vi "Matches.vi"(8 "error in (no error)":errorcluster, 10 "Actual":variant, 11 "Collection Is Empty in":refnum<class "Collection Is Empty.lvclass">) -> (0 "error out":errorcluster, 2 "Result":bool, 3 "Collection Is Empty out":refnum<class "Collection Is Empty.lvclass">)   [LabVIEW 2017, in "Transparent Assertions.lvlib" / "Collection Is Empty.lvclass"]
doc: "Evaluates the constraint for <B>Actual</B>. Returns true if the constraint is met."
uses:
  Collection Is Empty.lvclass
  Transparent Assertions.lvlib
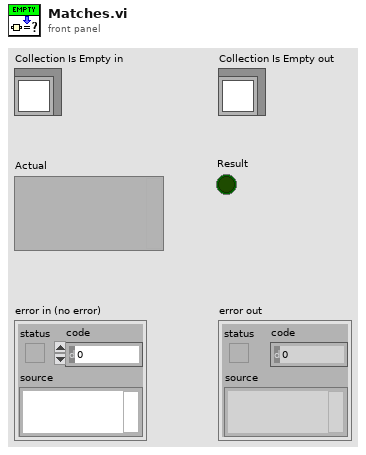
[diagram p1: front panel]
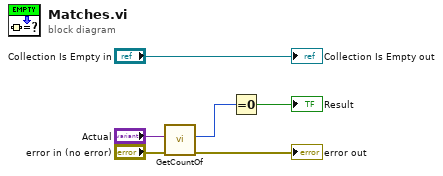
[diagram p0: block diagram]
diagram:
  n1 = call "GetCountOf.vi"("error in (no error)"="error in (no error)", "Countable"="Actual") -> ("error out"=→"error out":errorcluster, "Count"=w1:i32)  [unwired: 8 in]
  n2 = Equal To 0?(x=w1) -> (x = 0?=→"Result":bool)
  "Collection Is Empty out" <- "Collection Is Empty in"
